vi "Close Connection.vi"(8 "error in (no error)":errorcluster, 11 "RemoteControl.STM in":refnum<class "RemoteControl.STM.lvclass">) -> (0 "error out":errorcluster, 3 "RemoteControl.STM out":refnum<class "RemoteControl.STM.lvclass">)   [LabVIEW 2016, in "RemoteControl.STM.lvclass"]
uses:
  RemoteControl.STM.lvclass
  <vilib>/NI/STM/TCP/TCP Connection Info.ctl
  <vilib>/NI/STM/SubVIs/MetaDataElement.ctl
  <vilib>/NI/STM/Connection Manager/TCP/TCP Connection Method.ctl
  RemoteControl.STM.lvclass/RemoteControl.STM.ctl
  <vilib>/NI/STM/TCP/Get Connection Reference (TCP).vi
  <vilib>/NI/STM/NI STM.lvlib
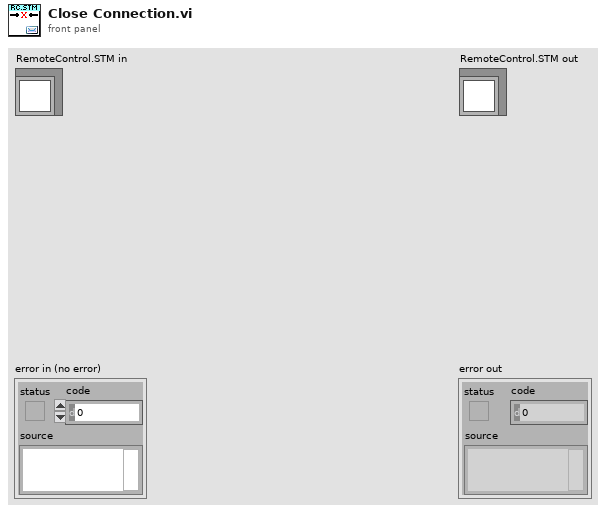
[diagram p1: front panel]
types:
  T1 = typedef "NI STM.lvlib/TCP Connection Method.ctl" = enum16{"Initialize", "Add Connection", "Set Properties", "Get Connection(s)", "Remove Connection", "Remove All Connections", "Get Connection Count"}
  T2 = typedef "NI STM.lvlib/TCP Connection Info.ctl" = cluster{"connection ID":refnum<k5>, "meta data":T3[]}
  T3 = typedef "NI STM.lvlib/MetaDataElement.ctl" = string
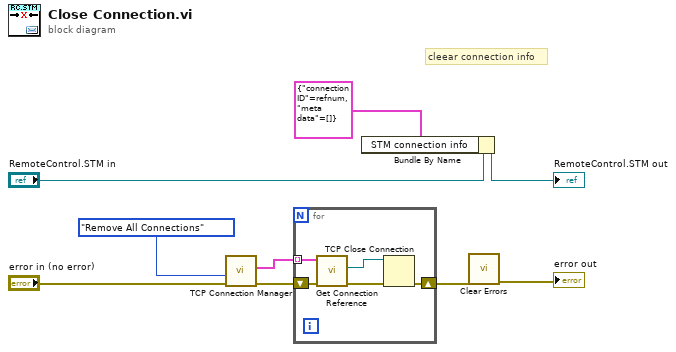
[diagram p0: block diagram]
diagram:
  # "cleear connection info"
  n1 = call <vilib>:"TCP Connection Manager.vi"("error in"="error in (no error)", "method"=TCP_Connection_Method."Remove All Connections") -> ("error out"=w3:errorcluster, "all connections"=w2:T2[])  [unwired: 4 in, 4 out]
  n2 = for {
    tunnel: w2 -> [w11] mode=indexing
    shift-right: [w10] -> w1
    shift-left: w3 -> [w12]
    n3 = call-poly <vilib>:"Get Connection Reference.vi"("error in"=w12, "connection info in"=w11) -> ("error out"=w13:errorcluster, "connection ID out"=w14:refnum<k5>)  [unwired: 7 in, 1 out]
    n4 = TCP Close Connection(connection ID=w14, error in (no error)=w13) -> (error out=w10:errorcluster)  [unwired: 1 in, 1 out]
  }
  n5 = Bundle By Name(cluster="RemoteControl.STM in", "STM connection info"=T2 {"connection ID"=refnum, "meta data"=[]}) -> (→"RemoteControl.STM out":refnum<class "RemoteControl.STM.lvclass">)
  n6 = call <vilib>:"Clear Errors.vi"("error in (no error)"=w1) -> ("error out"=→"error out":errorcluster)  [unwired: 5 in, 1 out]
